vi "encodeStream.vi"(8 "error in (no error)":errorcluster, 11 "tBSONJavaScript in":refnum<class "tBSONJavaScript.lvclass">) -> (0 "error out":errorcluster, 2 "Byte Array":u8[](array[numeric]), 3 "tBSONJavaScript out":refnum<class "tBSONJavaScript.lvclass">)   [LabVIEW 2013, in "BSON.lvlib" / "tBSONJavaScript.lvclass"]
uses:
  tBSONJavaScript.lvclass
  tBSONElement/tBSONElement.lvclass
  getScript.vi
  BSON.lvlib
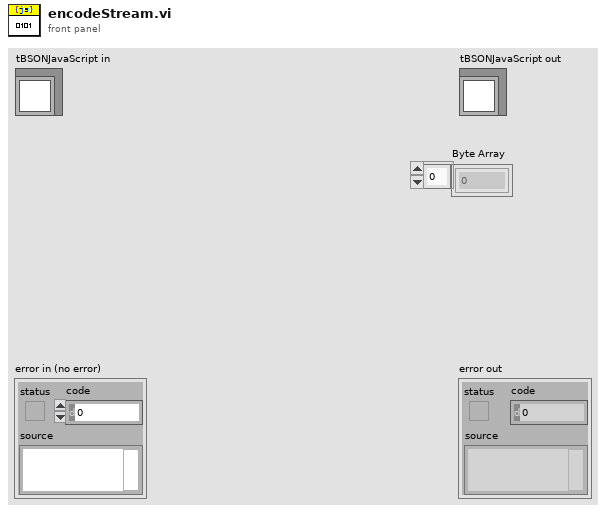
[diagram p1: front panel]
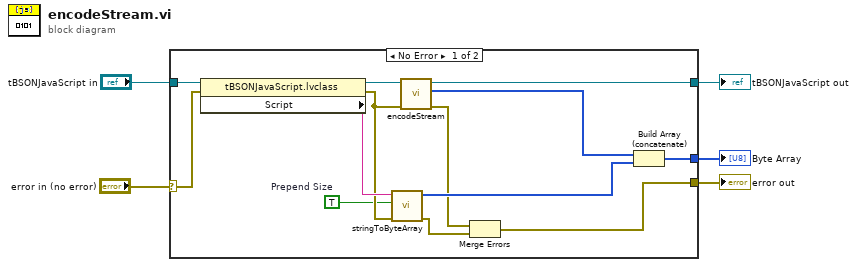
[diagram p0: block diagram]
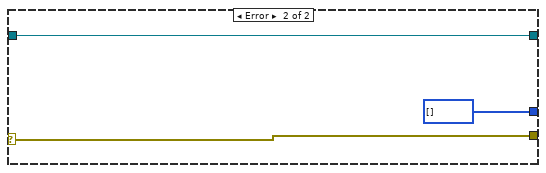
[diagram p2: hidden frame]
diagram:
  n1 = case shown="No Error" "error in (no error)" {
    selector: "error in (no error)" -> [w17 w20]
    tunnel: "tBSONJavaScript in" -> [w18 w21]
    tunnel: [w9 w21] -> w3
    tunnel: [w7 w20] -> w1
    tunnel: [w16 u8[] []] -> w2
    frame No Error {
      w6 = TRUE  # Prepend Size
      n2 = property class="tBSONJavaScript.lvclass"(reference=w18, error in=w17) -> (reference out=w12:refnum<class "tBSONJavaScript.lvclass">, error out=w11:errorcluster, "Script"=w15:string)
      n3 = call "stringToByteArray.vi"("error in (no error)"=w11, "Prepend Size"=w6, "String"=w15) -> ("error out"=w14:errorcluster, "byte array"=w13:u8[])  [unwired: 7 in]
      n4 = call-parent "encodeStream.vi"("error in (no error)"=w11, "tBSONElement in"=w12) -> ("error out"=w8:errorcluster, "Byte Array"=w10:u8[], "tBSONElement out"=w9:refnum<class "tBSONJavaScript.lvclass">)  [unwired: 7 in]
      n5 = Merge Errors(w8, w14) -> (w7:errorcluster)
      n6 = Build Array (concatenate)(w10, w13) -> (w16:u8[])
    }
    frame Error {
    }
  }
  "error out" <- w1
  "tBSONJavaScript out" <- w3
  "Byte Array" <- w2
